vi "Quality of Run Check.vi"(8 "error in (no error)":errorcluster, 11 "Monkey in":refnum<class "Monkey.lvclass">=refnum) -> (0 "error out":errorcluster, 2 "Check Result":T1, 3 "Monkey out":refnum<class "Monkey.lvclass">)   [LabVIEW 2020, in "CIRCUS_uServices.lvlib" / "Monkey.lvlib" / "Monkey.lvclass"]
uses:
  Monkey.lvclass
  Run Utilities/TypeDefs/Return Code.ctl
  Run Utilities/Run Utilities.lvlib
  Run Utilities/TypeDefs/DAQ Control.ctl
  Analysis Framework/Analysis Framework.lvclass
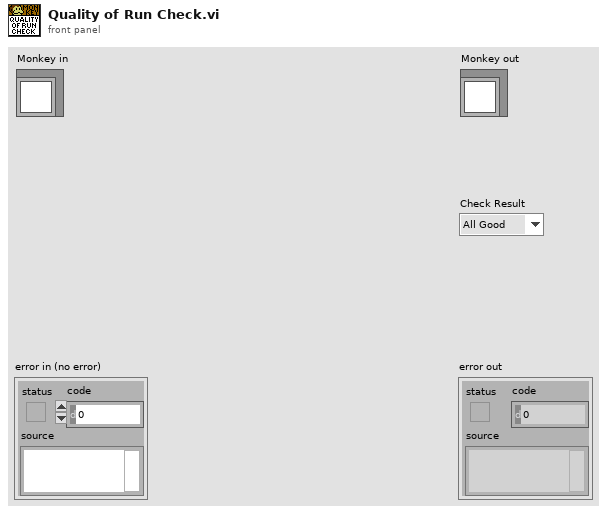
[diagram p1: front panel]
types:
  T1 = typedef "CIRCUS_uServices.lvlib/Run Utilities.lvlib/Return Code.ctl" = enum16{"All Good", "Retry", "Skip", "Skip All", "ABORT"}
  T2 = typedef "CIRCUS_uServices.lvlib/Run Utilities.lvlib/DAQ Control.ctl" = enum16{"On", "Off", "External"}
  T3 = cluster{"Name":string, "Comparison":string, "Value":string}[]
  T4 = typedef "CIRCUS_uServices.lvlib/Analysis Framework.lvclass/Name with value pair.ctl" = cluster{"Name":string, "Value":string}
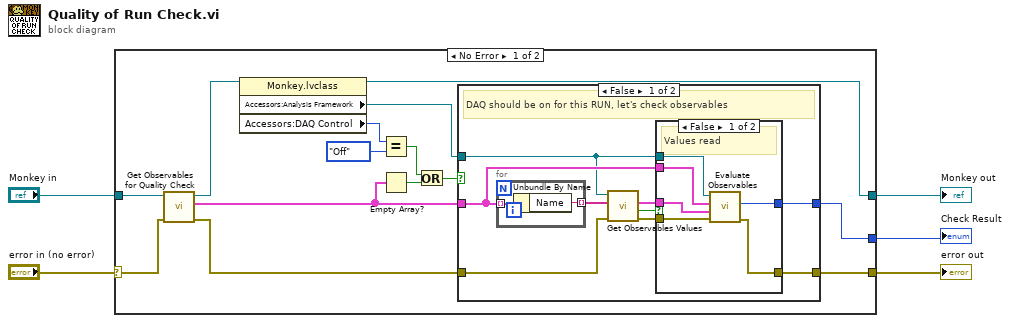
[diagram p0: block diagram]
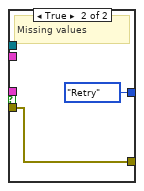
[diagram p2: hidden frame]
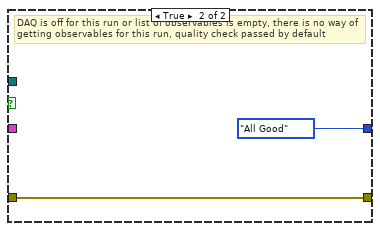
[diagram p3: hidden frame]
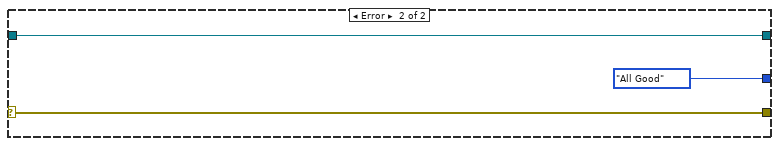
[diagram p4: hidden frame]
diagram:
  n1 = case shown="No Error" "error in (no error)" {
    selector: "error in (no error)" -> [w16 w43]
    tunnel: [w6 w43] -> w4
    tunnel: [w7 w42] -> w2
    tunnel: "Monkey in" -> [w14 w42]
    tunnel: [w8 Return_Code."All Good" ("f")] -> w1
    frame No Error {
      n2 = call-dynamic "Get Observables for Quality Check.vi"("error in (no error)"=w16, "Monkey in"=w14) -> ("error out"=w13:errorcluster, "Obsv to check"=w19:T3, "Monkey out"=w17:refnum<class "Monkey.lvclass">)  [unwired: 7 in]
      n3 = property class="Monkey.lvclass"(reference=w17) -> (reference out=w7:refnum<class "Monkey.lvclass">, "Accessors:Analysis Framework"=w9:refnum<class "Analysis Framework.lvclass">, "Accessors:DAQ Control"=w12:T2)  [unwired: 1 in, 1 out]
      n4 = Equal?(x=w12, y=DAQ_Control."Off") -> (x = y?=w10:bool)
      n5 = Empty Array?(array=w19) -> (empty?=w11:bool)
      n6 = Or(x=w10, y=w11) -> (x .or. y?=w18:bool)
      n7 = case shown="False" w18 {
        tunnel: [w22 Return_Code."All Good" ("f")] -> w8
        tunnel: [w20 w39] -> w6
        tunnel: w13 -> [w28 w39]
        tunnel: w19 -> [w24 _]
        tunnel: w9 -> [w23 _]
        frame False {
          # "DAQ should be on for this RUN, let's check observables"
          n8 = for {
            tunnel: w24 -> [w38] mode=indexing
            tunnel: [w37] -> w27 mode=indexing
            n9 = Unbundle By Name(w38) -> ("Name"=w37:string)
          }
          n10 = call-dynamic "Get Observables Values.vi"("error in (no error)"=w28, "Observables"=w27, "Analysis Framework in"=w23) -> ("error out"=w26:errorcluster, "Missing values"=w21:bool, "Observables with values"=w25:T4[])  [unwired: 5 in, 1 out]
          n11 = case shown="False" w21 {
            tunnel: w26 -> [w34 w35]
            tunnel: w25 -> [w33 _]
            tunnel: w24 -> [w32 _]
            tunnel: w23 -> [w31 _]
            tunnel: [w30 Return_Code."Retry" ("Evaluation")] -> w22
            tunnel: [w29 w35] -> w20
            frame False {
              # "Values read"
              n12 = call-dynamic "Evaluate Observables.vi"("error in (no error)"=w34, "Observables with values"=w33, "Obsv to check"=w32, "Analysis Framework in"=w31) -> ("error out"=w29:errorcluster, "Evaluation"=w30:T1)  [unwired: 5 in, 1 out]
            }
            frame True {
              # "Missing values"
            }
          }
        }
        frame True {
          # "DAQ is off for this run or list of observables is empty, there is no way of getting observables for this run, quality check passed by default"
        }
      }
    }
    frame Error {
    }
  }
  "error out" <- w4
  "Monkey out" <- w2
  "Check Result" <- w1
